vi "Main.vi"() -> ()   [LabVIEW 2017, in "Composition.Tests.lvlib"]
uses:
  Composition.Tests.lvlib
  2d79373b-df2c-414a-af86-da62c28e88f5.vi
  e4ca86ee-a803-44c1-bdc9-63bf4b454cd2.vi
  Composition/Get ClassName From Flattened Object.vi
  <vilib>/Utility/LVClass/Qualified Name Array To Single String.vi
  Composition/Composition.lvlib
  Classes/Aggregate/Aggregate.lvclass
  Classes/String/String.lvclass
  Classes/Child/Child.lvclass
  <vilib>/addons/_JKI Toolkits/Caraya/classes/Assert/Assert.lvclass
  <vilib>/addons/_JKI Toolkits/Caraya/classes/Test/Test.lvclass
panel:
  out "error out":errorcluster
  # "This application performs various runtime tests to verify that the functions in this library do not depend on edit-time behavior."
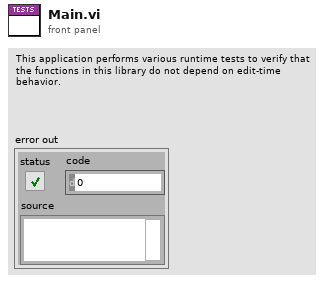
[diagram p1: front panel]
types:
  T1 = cluster{string, bool, dbl, dbl[], cluster{string, bool}}
  T2 = cluster{"String out":refnum<class "String.lvclass">, "Child out":refnum<class "Child.lvclass">}
  T3 = cluster{"Major":u16, "Minor":u16, "Fix":u16, "Build":u16}[]
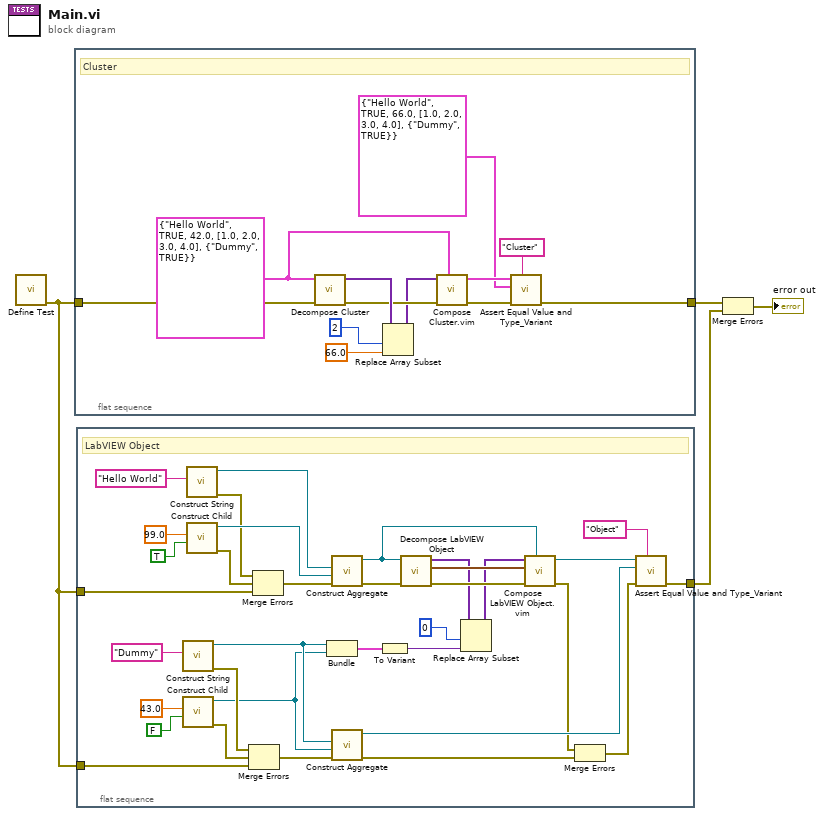
[diagram p0: block diagram]
diagram:
  n1 = call <vilib>:"Define Test.vi"() -> ("error out"=w1:errorcluster)  [unwired: 10 in, 1 out]
  n2 = flat-sequence {
    tunnel: [w9] -> w4
    tunnel: w1 -> [w6]
    frame #0 {
      w10 = T1 {"Hello World", TRUE, 42.0, [1.0, 2.0, 3.0, 4.0], {"Dummy", TRUE}}
      # "Cluster"
      n3 = call "Decompose Cluster.vi"("error in (no error)"=w6, "Cluster"=w10) -> ("error out"=w14:errorcluster, "Cluster Elements"=w15:variant[])  [unwired: 8 in]
      n4 = Replace Array Subset(array=w15, new element=66.0, index=2) -> (w13:variant[])
      n5 = call "Compose Cluster.vim"("Type"=w10, "error in"=w14, "Elements"=w13) -> ("error out"=w16:errorcluster, "Cluster"=w8:T1)  [unwired: 7 in]
      n6 = call <vilib>:"Assert Equal Value and Type_Variant.vi"("Label"="Cluster", "error in (no error)"=w16, "Y"=T1 {"Hello World", TRUE, 66.0, [1.0, 2.0, 3.0, 4.0], {"Dummy", TRUE}}, "X"=w8) -> ("error out"=w9:errorcluster)  [unwired: 6 in, 1 out]
    }
  }
  n7 = flat-sequence {
    tunnel: [w25] -> w2
    tunnel: w1 -> [w19]
    tunnel: w1 -> [w18]
    frame #0 {
      # "LabVIEW Object"
      n8 = call "Construct String.vi"("String"="Dummy") -> ("error out"=w35:errorcluster, "String out"=w32:refnum<class "String.lvclass">)  [unwired: 9 in]
      n9 = call "Construct Child.vi"("Ignored"=FALSE, "Offset"=43.0) -> ("error out"=w36:errorcluster, "Child out"=w31:refnum<class "Child.lvclass">)  [unwired: 8 in]
      n10 = call "Construct String.vi"("String"="Hello World") -> ("error out"=w46:errorcluster, "String out"=w50:refnum<class "String.lvclass">)  [unwired: 9 in]
      n11 = call "Construct Child.vi"("Ignored"=TRUE, "Offset"=99.0) -> ("error out"=w45:errorcluster, "Child out"=w49:refnum<class "Child.lvclass">)  [unwired: 8 in]
      n12 = Merge Errors(w35, w36, w18) -> (w34:errorcluster)
      n13 = Merge Errors(w46, w45, w19) -> (w48:errorcluster)
      n14 = Bundle("String out"=w32, "Child out"=w31) -> (w30:T2)  [unwired: 1 in]
      n15 = call "Construct Aggregate.vi"("error in (no error)"=w48, "Reflection.Tests.lvlib:Child.lvclass"=w49, "Reflection.Tests.lvlib:String.lvclass"=w50) -> ("error out"=w47:errorcluster, "Aggregate out"=w40:refnum<class "Aggregate.lvclass">)  [unwired: 7 in]
      n16 = call "Construct Aggregate.vi"("error in (no error)"=w34, "Reflection.Tests.lvlib:Child.lvclass"=w31, "Reflection.Tests.lvlib:String.lvclass"=w32) -> ("error out"=w21:errorcluster, "Aggregate out"=w24:refnum<class "Aggregate.lvclass">)  [unwired: 7 in]
      n17 = To Variant(anything=w30) -> (Variant=w26:variant)
      n18 = call "Decompose LabVIEW Object.vi"("error in (no error)"=w47, "LabVIEW Object"=w40) -> ("error out"=w41:errorcluster, "Library Versions"=w33:T3, "Private Data Clusters"=w29:variant[])  [unwired: 6 in, 1 out]
      n19 = Replace Array Subset(array=w29, new element=w26, index=0) -> (w28:variant[])
      n20 = call "Compose LabVIEW Object.vim"("Type"=w40, "error in (no error)"=w41, "Library Versions"=w33, "Private Data Clusters"=w28) -> ("error out"=w22:errorcluster, "LabVIEW Object"=w23:refnum<class "Aggregate.lvclass">)  [unwired: 6 in]
      n21 = Merge Errors(w22, w21) -> (w20:errorcluster)
      n22 = call <vilib>:"Assert Equal Value and Type_Variant.vi"("Label"="Object", "error in (no error)"=w20, "Y"=w24, "X"=w23) -> ("error out"=w25:errorcluster)  [unwired: 6 in, 1 out]
    }
  }
  n23 = Merge Errors(w4, w2) -> (→"error out":errorcluster)
